vi "VI Tree.vi"   [LabVIEW 2009, in "Agilent 8000 Series.lvlib"]
doc: "This is the instrument driver for the Agilent 8000 and 80000 Series Oscilloscopes. The VI Tree displays all the user-callable VIs of the instrument driver in an organized table."
uses:
  Agilent 8000 Series.lvlib
  Configure/Configure Math (Unary Operation).vi
  Configure/Configure Measurement Characteristics (Eye Pattern).vi
  Data/Low Level/Fetch (Waveform).vi
  Configure/Configure Measurement Histogram (More).vi
  Configure/Configure Measurement Trend (More).vi
  Configure/Configure Jitter Spectrum (More).vi
  Data/Low Level/Fetch Measurement (More).vi
  Data/Read (Single Waveform).vi
  Configure/Configure Trigger (Pattern).vi
  Data/Read Measurement (Data Rate-Unit Interval).vi
panel:
  # "(c) 2008-2015 National Instruments.  ALL RIGHTS RESERVED."
  # "SEE DIAGRAM\nFOR VI TREE."
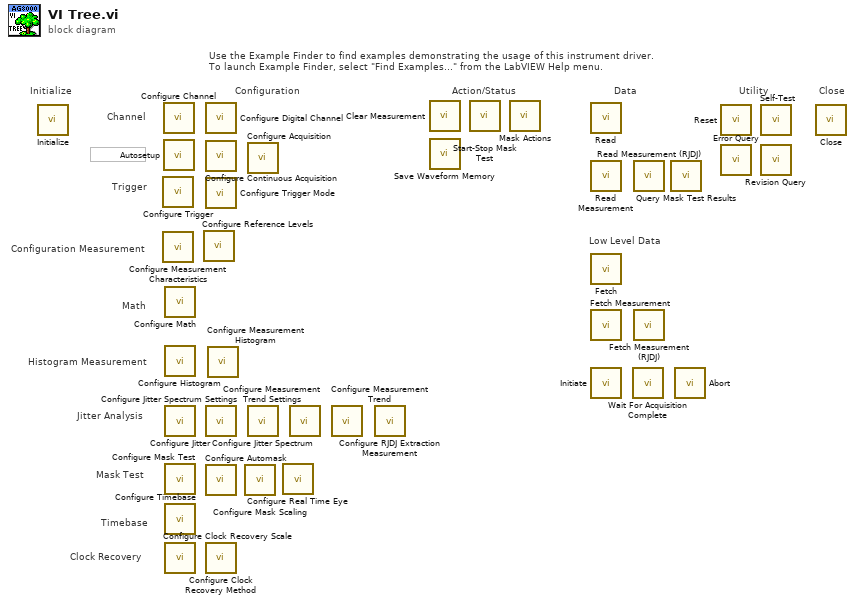
[diagram p0: block diagram]
diagram:
  # "Clock Recovery"
  # "Mask Test"
  # "Jitter Analysis"
  # "Histogram Measurement"
  # "Math"
  # "Trigger"
  # "Configuration Measurement"
  # "Timebase"
  # "Channel"
  # "Low Level Data"
  # "Action/Status"
  # "Use the Example Finder to find examples demonstrating the usage of this instrument driver.\nTo launch Example Finder, select \"Find Examples...\" from the LabVIEW Help menu."
  # "Configuration"
  # "Utility"
  # "Data"
  # "Close"
  # "Initialize"
  n1 = call "Initialize.vi"() -> ()  [unwired: 10 in, 2 out]
  n2 = call-poly "Configure Trigger.vi"() -> ()  [unwired: 14 in, 2 out]
  n3 = call-poly "Configure Measurement Characteristics.vi"() -> ()  [unwired: 14 in, 2 out]
  n4 = call "Configure Channel.vi"() -> ()  [unwired: 14 in, 2 out]
  n5 = call "Autosetup.vi"() -> ()  [unwired: 10 in, 2 out]
  n6 = call-poly "Configure Math.vi"() -> ()  [unwired: 14 in, 2 out]
  n7 = call "Configure Histogram.vi"() -> ()  [unwired: 14 in, 2 out]
  n8 = call "Configure Jitter.vi"() -> ()  [unwired: 10 in, 2 out]
  n9 = call "Configure Mask Test.vi"() -> ()  [unwired: 14 in, 2 out]
  n10 = call "Configure Timebase.vi"() -> ()  [unwired: 10 in, 2 out]
  n11 = call "Configure Clock Recovery Scale.vi"() -> ()  [unwired: 10 in, 2 out]
  n12 = call "Configure Reference Levels.vi"() -> ()  [unwired: 10 in, 2 out]
  n13 = call "Configure Digital Channel.vi"() -> ()  [unwired: 10 in, 2 out]
  n14 = call "Configure Continuous Acquisition.vi"() -> ()  [unwired: 10 in, 2 out]
  n15 = call "Configure Trigger Mode.vi"() -> ()  [unwired: 10 in, 2 out]
  n16 = call "Configure Jitter Spectrum Settings.vi"() -> ()  [unwired: 14 in, 2 out]
  n17 = call "Configure Automask.vi"() -> ()  [unwired: 10 in, 2 out]
  n18 = call "Configure Clock Recovery Method.vi"() -> ()  [unwired: 14 in, 2 out]
  n19 = call-poly "Configure Measurement Histogram.vi"() -> ()  [unwired: 14 in, 2 out]
  n20 = call "Configure Mask Scaling.vi"() -> ()  [unwired: 10 in, 2 out]
  n21 = call "Configure Acquisition.vi"() -> ()  [unwired: 14 in, 2 out]
  n22 = call-poly "Configure Jitter Spectrum.vi"() -> ()  [unwired: 14 in, 2 out]
  n23 = call "Configure Real Time Eye.vi"() -> ()  [unwired: 10 in, 2 out]
  n24 = call "Configure Measurement Trend Settings.vi"() -> ()  [unwired: 14 in, 2 out]
  n25 = call-poly "Configure Measurement Trend.vi"() -> ()  [unwired: 14 in, 2 out]
  n26 = call "Configure RJDJ Extraction Measurement.vi"() -> ()  [unwired: 14 in, 2 out]
  n27 = call "Clear Measurement.vi"() -> ()  [unwired: 10 in, 2 out]
  n28 = call "Save Waveform Memory.vi"() -> ()  [unwired: 10 in, 2 out]
  n29 = call "Start-Stop Mask Test.vi"() -> ()  [unwired: 10 in, 2 out]
  n30 = call "Mask Actions.vi"() -> ()  [unwired: 10 in, 2 out]
  n31 = call-poly "Read.vi"() -> ()  [unwired: 9 in, 3 out]
  n32 = call-poly "Read Measurement.vi"() -> ()  [unwired: 13 in, 3 out]
  n33 = call-poly "Fetch.vi"() -> ()  [unwired: 9 in, 3 out]
  n34 = call-poly "Fetch Measurement.vi"() -> ()  [unwired: 13 in, 3 out]
  n35 = call "Initiate.vi"() -> ()  [unwired: 10 in, 2 out]
  n36 = call "Wait For Acquisition Complete.vi"() -> ()  [unwired: 10 in, 2 out]
  n37 = call "Read Measurement (RJDJ).vi"() -> ()  [unwired: 7 in, 9 out]
  n38 = call "Fetch Measurement (RJDJ).vi"() -> ()  [unwired: 7 in, 9 out]
  n39 = call "Query Mask Test Results.vi"() -> ()  [unwired: 6 in, 6 out]
  n40 = call "Abort.vi"() -> ()  [unwired: 10 in, 2 out]
  n41 = call "Reset.vi"() -> ()  [unwired: 10 in, 2 out]
  n42 = call "Error Query.vi"() -> ()  [unwired: 8 in, 4 out]
  n43 = call "Self-Test.vi"() -> ()  [unwired: 8 in, 4 out]
  n44 = call "Revision Query.vi"() -> ()  [unwired: 8 in, 4 out]
  n45 = call "Close.vi"() -> ()  [unwired: 11 in, 1 out]
